vi "Get Video Mode.vi"(8 "error in (no error)":errorcluster, 11 "VISA resource name":refnum<visa-resource-name>) -> (0 "error out":errorcluster, 1 "Video Line Marker":i32, 2 "Video Format":i32, 3 "VISA resource name out":refnum<visa-resource-name>)   [LabVIEW 2013, in "Fluke 5XXX Series Multicalibrators.lvlib"]
doc: "This VI returns the format of Video scope mode and returns the Video mode line marker location.\n\nNote:\n\nThis VI is available only for instrument models 5500A and 5520A with oscilloscope option SC600 (SC1100)."
uses:
  Fluke 5XXX Series Multicalibrators.lvlib
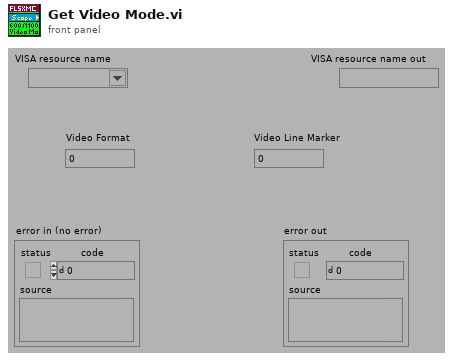
[diagram p1: front panel]
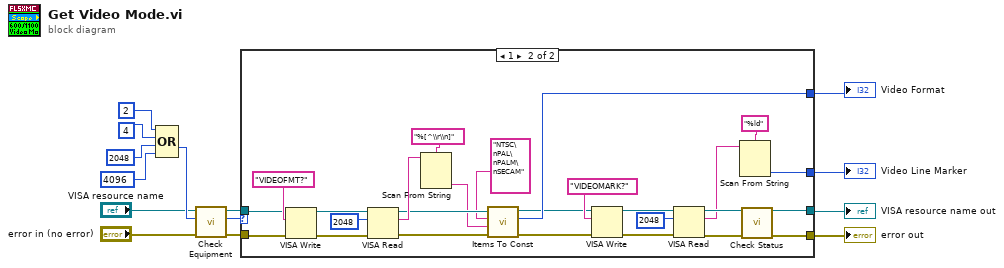
[diagram p0: block diagram]
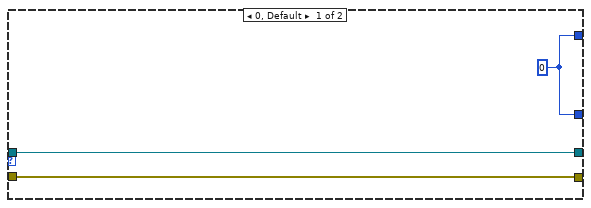
[diagram p2: hidden frame]
diagram:
  n1 = Compound Arithmetic op=OR(2 ("Numeric"), 4 ("Numeric"), 2048 ("Numeric"), 4096 ("Numeric")) -> (w7:i32)
  n2 = call "Check Equipment.vi"("error in (no error)"="error in (no error)", "Bit Mask"=w7, "VISA resource name"="VISA resource name") -> ("error out"=w14:errorcluster, "Present?"=w13:u32, "VISA resource name out"=w12:refnum<visa-resource-name>)  [unwired: 6 in]
  n3 = case shown="1" w13 {
    tunnel: [w17 w37] -> w4
    tunnel: [w16 w36] -> w3
    tunnel: w14 -> [w17 w39]
    tunnel: w12 -> [w16 w38]
    tunnel: [w15 w30] -> w1
    tunnel: [w15 w19] -> w2
    frame 0, Default {
      w15 = 0
    }
    frame 1 {
      n4 = VISA Write(VISA resource name=w38, write buffer="VIDEOFMT?", error in (no error)=w39) -> (VISA resource name out=w42:refnum<visa-resource-name>, error out=w41:errorcluster)  [unwired: 1 out]
      n5 = VISA Read(VISA resource name=w42, byte count=u32 2048 ("byte count (0)"), error in (no error)=w41) -> (VISA resource name out=w32:refnum<visa-resource-name>, read buffer=w34:string, error out=w33:errorcluster)  [unwired: 1 out]
      n6 = Scan From String(format string="%[^\\r\\n]", input string=w34) -> (output 1=w31:string)  [unwired: 3 in, 3 out]
      n7 = call "Items To Const.vi"("error in (no error)"=w33, "String Item"=w31, "Multi-Line String"="NTSC\nPAL\nPALM\nSECAM", "VISA resource name"=w32) -> ("error out"=w22:errorcluster, "Index"=w30:i32, "VISA resource name out"=w23:refnum<visa-resource-name>)  [unwired: 5 in]
      n8 = VISA Write(VISA resource name=w23, write buffer="VIDEOMARK?", error in (no error)=w22) -> (VISA resource name out=w28:refnum<visa-resource-name>, error out=w26:errorcluster)  [unwired: 1 out]
      n9 = VISA Read(VISA resource name=w28, byte count=u32 2048 ("byte count (0)"), error in (no error)=w26) -> (VISA resource name out=w24:refnum<visa-resource-name>, read buffer=w20:string, error out=w25:errorcluster)  [unwired: 1 out]
      n10 = Scan From String(format string="%ld", input string=w20) -> (output 1=w19:i32)  [unwired: 3 in, 3 out]
      n11 = call "Check Status.vi"("VISA resource name"=w24, "error in (no error)"=w25) -> ("VISA resource name out"=w36:refnum<visa-resource-name>, "error out"=w37:errorcluster)  [unwired: 12 in]
    }
  }
  "Video Format" <- w1
  "Video Line Marker" <- w2
  "VISA resource name out" <- w3
  "error out" <- w4
